vi "Create Temp Build Spec File Name.vi"(0 "Export":refnum<class "Export.lvclass">) -> (4 "Export":refnum<class "Export.lvclass">, 6 "Temporary build spec Path":path, 15 "error IO":errorcluster)   [LabVIEW 2017, in "CL_G3_VIComponentBuilder.lvlib" / "Export.lvclass"]
doc: "Creates a temporary name for the build specification. This name is typlicaly used during build to create a copy of the build spec while it is being edited. The temp copy overwrites the original during commit."
uses:
  Export.lvclass
  Export.lvclass/Export.ctl
  Accessors/Read Export Build Specification.vi
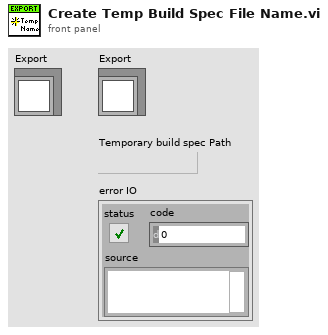
[diagram p1: front panel]
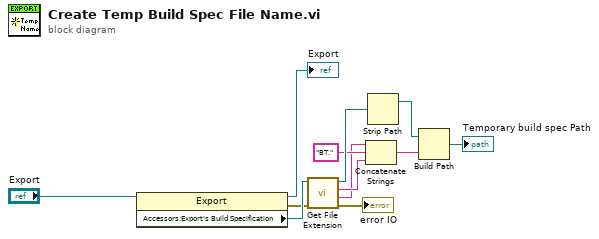
[diagram p0: block diagram]
diagram:
  n1 = property class="Export"(reference="Export") -> (reference out=→"Export":refnum<class "Export.lvclass">, error out=w1:errorcluster, "Accessors:Export's Build Specification"=w11:path)  [unwired: 1 in]
  n2 = call <vilib>:"Get File Extension.vi"("error in (no error)"=w1, "file"=w11) -> ("error out"=→"error IO":errorcluster, "filename without extension"=w2:string, "lowercase file extension"=w4:string, "dup file"=w5:path)  [unwired: 5 in, 1 out]
  n3 = Concatenate Strings(w2, "BT." ("string"), w4) -> (w7:string)
  n4 = Strip Path(path=w5) -> (stripped path=w6:path)  [unwired: 1 out]
  n5 = Build Path(base path=w6, name or relative path=w7) -> (appended path=→"Temporary build spec Path":path)
